vi "Read PV.vi"(8 "error in (no error)":errorcluster, 11 "CS++PVUpdate Msg in":refnum<class "CS++PVUpdate Msg.lvclass">) -> (0 "error out":errorcluster, 2 "PV":refnum<class "PV.lvclass">, 3 "CS++PVUpdate Msg out":refnum<class "CS++PVUpdate Msg.lvclass">)   [LabVIEW 2012, in "CS++PVMonitor.lvlib" / "CS++PVUpdate Msg.lvclass"]
uses:
  CS++PVUpdate Msg.lvclass
  Classes/CS++ProcessVariables/ProcessVariable/PV.lvclass
  CS++PVUpdate Msg.lvclass/CS++PVUpdate Msg.ctl
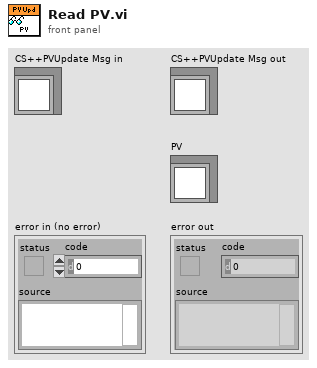
[diagram p1: front panel]
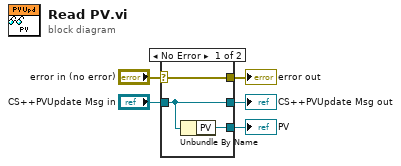
[diagram p0: block diagram]
diagram:
  n1 = case shown="No Error" "error in (no error)" {
    selector: "error in (no error)" -> [w8 w9]
    tunnel: [w8 w9] -> w4
    tunnel: [w7 w10] -> w2
    tunnel: "CS++PVUpdate Msg in" -> [w7 w10]
    tunnel: [w6 _] -> w1
    frame No Error {
      n2 = Unbundle By Name(w7) -> ("PV"=w6:refnum<class "PV.lvclass">)
    }
    frame Error {
    }
  }
  "error out" <- w4
  "CS++PVUpdate Msg out" <- w2
  "PV" <- w1
